vi "Config Read Sequence Steps.vi"(8 "Error In":errorcluster, 9 "Base Path":path=path "C:/Labview Code/System/Part Configuration", 10 "Part Type":string, 11 "Station Name":string) -> (0 "Error Out":errorcluster, 2 "VI Names":string[](array[string]), 3 "Sequence Steps":string[](array[string]))   [LabVIEW 2018]
uses:
  <vilib>/Utility/config.llb/Read Key (String).vi
  <vilib>/Utility/config.llb/NI_LVConfig.lvlib
panel:
  out "All Keys":string[](array[string])
  out "All Sections":string[](array[string])
  # "6"
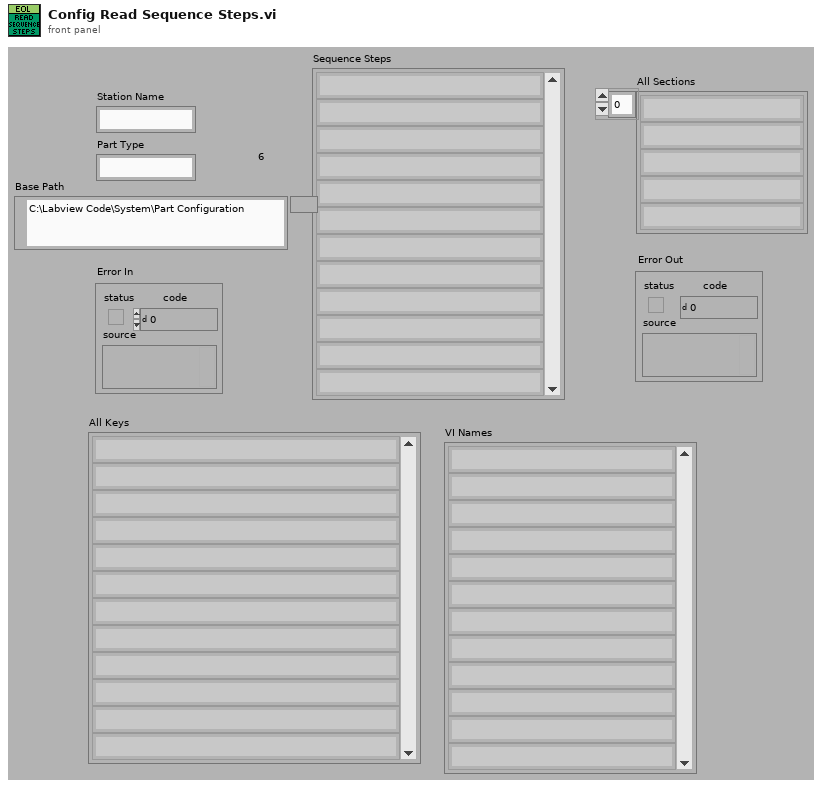
[diagram p1: front panel]
types:
  T1 = typedef "NI_LVConfig.lvlib/Config Data RefNum.ctl" = refnum<k1>
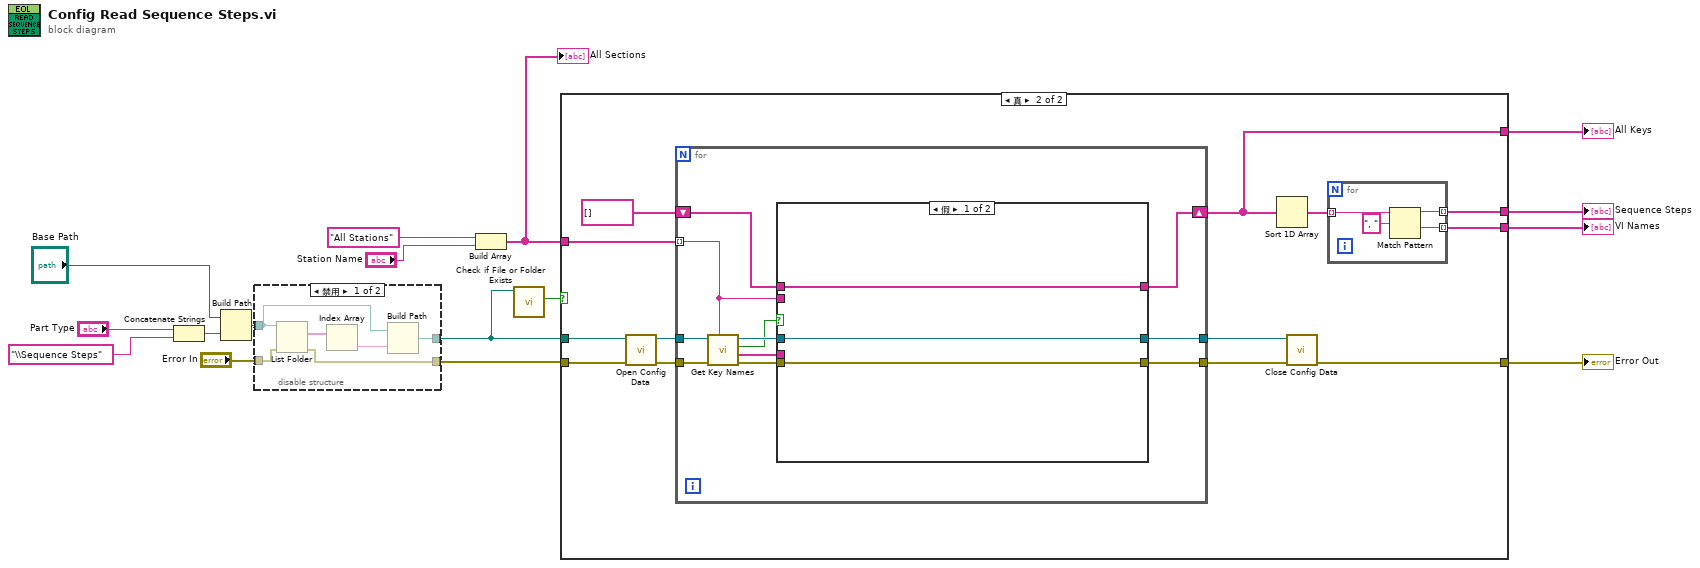
[diagram p0: block diagram]
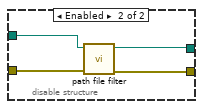
[diagram p2: hidden frame]
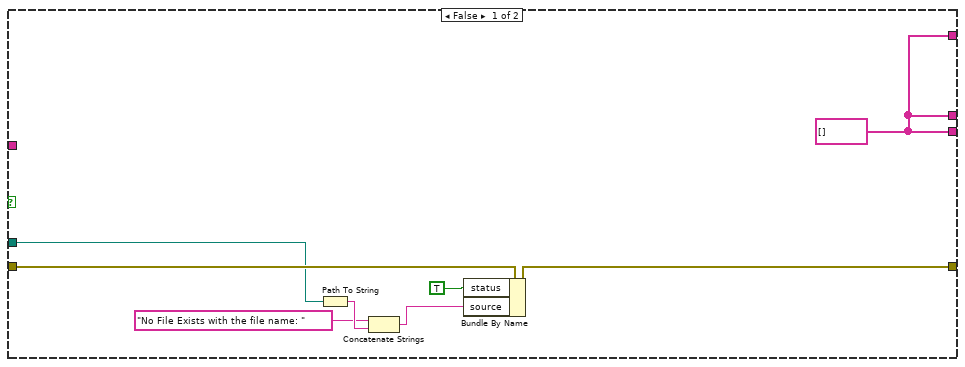
[diagram p3: hidden frame]
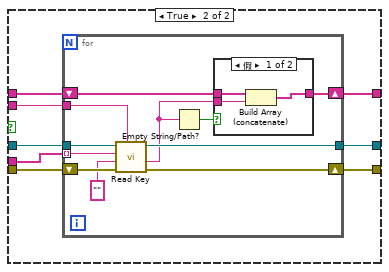
[diagram p4: hidden frame]
diagram:
  n1 = Concatenate Strings("Part Type", "\\Sequence Steps" ("string")) -> (w9:string)
  n2 = Build Path(base path="Base Path", name or relative path=w9) -> (appended path=w10:path)
  n3 = disable-structure shown="禁用" {
    disable-tunnel: w10 -> [w20 w26]
    disable-tunnel: [w19 w25] -> w4
    disable-tunnel: "Error In" -> [w18 w24]
    disable-tunnel: [w17 w23] -> w1
    frame Disabled {
      n4 = List Folder(path=w20, error in=w18) -> (filenames=w21:string[], error out=w17:errorcluster)  [unwired: 2 in, 2 out]
      n5 = Index Array(array=w21) -> (element=w22:string)  [unwired: 1 in]
      n6 = Build Path(base path=w20, name or relative path=w22) -> (appended path=w19:path)
    }
    frame Enabled {
      n7 = call "path file filter.vi"("Sys Error In"=w24, "path"=w26) -> ("错误输出"=w23:errorcluster, "File path"=w25:path)  [unwired: 8 in]
    }
  }
  n8 = Build Array("All Stations", "Station Name") -> (w11:string[])
  "All Sections" <- w11
  n9 = call <vilib>:"Check if File or Folder Exists.vi"("path"=w4) -> ("file or folder exists?"=w5:bool)  [unwired: 8 in, 2 out]
  n10 = case shown="真" w5 {
    tunnel: w4 -> [w27 w47]
    tunnel: [w32 w42] -> w16
    tunnel: w1 -> [w33 w41]
    tunnel: [w31 w40] -> w15
    tunnel: [w31 w39] -> w14
    tunnel: [w31 w37] -> w13
    tunnel: w11 -> [_ w36]
    frame False {
      w31 = string[] []
      n11 = Path To String(path=w27) -> (string=w30:string)
      n12 = Concatenate Strings("No File Exists with the file name: " ("string"), w30) -> (w28:string)
      n13 = Bundle By Name(cluster=w33, "status"=TRUE, "source"=w28) -> (w32:errorcluster)
    }
    frame True {
      n14 = call <vilib>:"Open Config Data.vi"("error in (no error)"=w41, "configuration file path"=w47) -> ("error out"=w45:errorcluster, "refnum"=w46:T1)  [unwired: 7 in, 1 out]
      n15 = for {
        tunnel: w46 -> [w62]
        tunnel: w45 -> [w61]
        tunnel: [w57] -> w44
        tunnel: [w56] -> w43
        tunnel: w36 -> [w55] mode=indexing
        shift-right: [w53] -> w37
        shift-left: string[] [] -> [w54]
        n16 = call <vilib>:"Get Key Names.vi"("section"=w55, "error in (no error)"=w61, "refnum"=w62) -> ("error out"=w60:errorcluster, "key names"=w52:string[], "section exists?"=w58:bool, "refnum out"=w59:T1)  [unwired: 5 in]
        n17 = case shown="假" w58 {
          tunnel: w52 -> [_ w73]
          tunnel: w60 -> [w65 w72]
          tunnel: w59 -> [w64 w71]
          tunnel: w55 -> [_ w70]
          tunnel: [w65 w69] -> w57
          tunnel: [w63 w68] -> w53
          tunnel: [w64 w67] -> w56
          tunnel: w54 -> [w63 w66]
          frame False {
          }
          frame True {
            n18 = for {
              tunnel: w73 -> [w82] mode=indexing
              tunnel: w71 -> [w84]
              tunnel: w70 -> [w83]
              shift-right: [w80] -> w69
              shift-left: w72 -> [w81]
              tunnel: [w78] -> w67
              shift-right: [w77] -> w68
              shift-left: w66 -> [w76]
              n19 = call-poly <vilib>:"Read Key.vi"("section"=w83, "error in (no error)"=w81, "default value"="", "key"=w82, "refnum"=w84) -> ("error out"=w80:errorcluster, "value"=w74:string, "refnum out"=w78:T1)  [unwired: 3 in, 1 out]
              n20 = Empty String/Path?(string/path=w74) -> (empty?=w75:bool)
              n21 = case shown="假" w75 {
                tunnel: w74 -> [w87 _]
                tunnel: [w86 w88] -> w77
                tunnel: w76 -> [w85 w88]
                frame False {
                  n22 = Build Array (concatenate)(w85, w87) -> (w86:string[])
                }
                frame True {
                }
              }
            }
          }
        }
      }
      n23 = Sort 1D Array(array=w37) -> (sorted array=w38:string[])
      n24 = call <vilib>:"Close Config Data.vi"("error in (no error)"=w44, "refnum"=w43) -> ("error out"=w42:errorcluster)  [unwired: 8 in, 1 out]
      n25 = for {
        tunnel: w38 -> [w51] mode=indexing
        tunnel: [w49] -> w39 mode=indexing
        tunnel: [w48] -> w40 mode=indexing
        n26 = Match Pattern(string=w51, regular expression=", ") -> (before substring=w49:string, after substring=w48:string)  [unwired: 1 in, 2 out]
      }
    }
  }
  "Sequence Steps" <- w14
  "Error Out" <- w16
  "VI Names" <- w15
  "All Keys" <- w13
